vi "Setup.vi"(8 "error in (no error)":errorcluster, 11 "Environment.LogFile in":refnum<class "Environment.LogFile.lvclass">) -> (0 "error out":errorcluster, 3 "Environment.LogFile out":refnum<class "Environment.LogFile.lvclass">)   [LabVIEW 2018, in "Environment.LogFile.lvclass"]
uses:
  Environment.LogFile.lvclass
panel:
  # "Connector Pane"
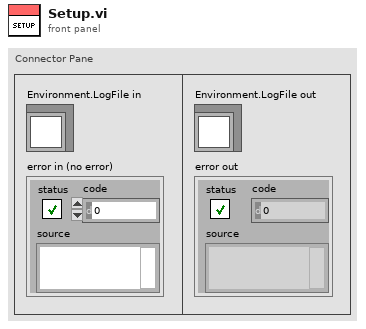
[diagram p1: front panel]
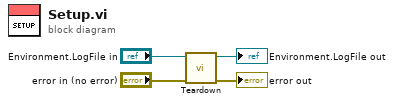
[diagram p0: block diagram]
diagram:
  n1 = call-dynamic "Teardown.vi"("error in (no error)"="error in (no error)", "Environment.LogFile in"="Environment.LogFile in") -> ("error out"=→"error out":errorcluster, "Environment.LogFile out"=→"Environment.LogFile out":refnum<class "Environment.LogFile.lvclass">)  [unwired: 8 in]
